vi "rszvl Configure Reference Oscillator.vi"(8 "error in (no error)":errorcluster, 10 "Reference (Internal)":i32(ring) items=["Internal", "External"], 11 "VISA resource name":refnum<visa-resource-name>) -> (0 "error out":errorcluster, 3 "VISA resource name out":refnum<visa-resource-name>)   [LabVIEW 2014]
doc: "This VI selects the source of the reference oscillator signal.\n\nAttribute(s):\nRSZVL_ATTR_ROSC_SOURCE\n\nRemote-control command(s):\n[SENSe<Ch>:]ROSCillator[:SOURce] INTernal | EXTernal"
uses:
  Instance           1 44Saved   rszvl Configure Reference Oscillator .vi
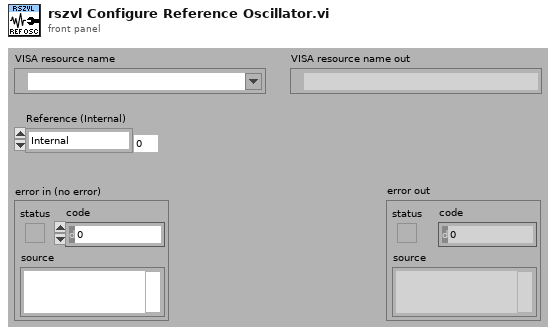
[diagram p1: front panel]
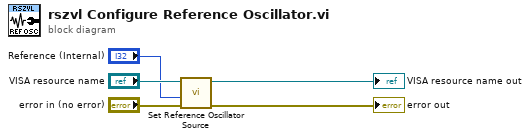
[diagram p0: block diagram]
diagram:
  n1 = call "Set Reference Oscillator Source"("error in (no error)"="error in (no error)", "Reference Oscillator Source (0 - SOUR_INT)"="Reference (Internal)", "instrument handle"="VISA resource name") -> ("error out"=→"error out":errorcluster, "instrument handle out"=→"VISA resource name out":refnum<visa-resource-name>)  [unwired: 7 in]
